vi "isMotorOn.vi"(1 "Device":refnum<k24>) -> (0 "isConnected":bool)   [LabVIEW 2014]
doc: "André Romero - 2017\nandretec@ifsc.usp.br"
uses:
  C:/UserLabs/Andre/LabView2014-32bits/kinesisTec/Kinesis/Thorlabs.MotionControl.TCube.DCServoCLI.dll
  Kinesis/Thorlabs.MotionControl.TCube.DCServoCLI.dll
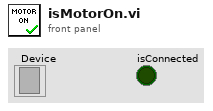
[diagram p1: front panel]
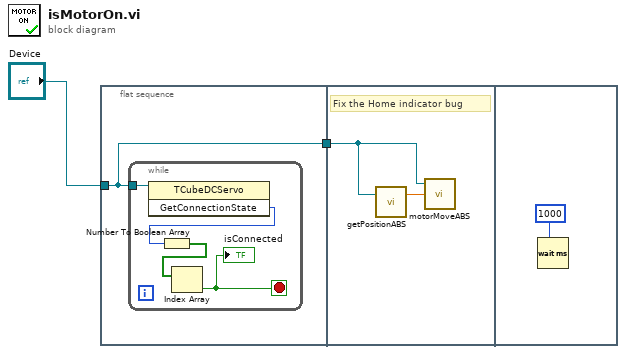
[diagram p0: block diagram]
diagram:
  n1 = flat-sequence {
    tunnel: "Device" -> [w3]
    tunnel: [w3] -> w1
    tunnel: w1 -> [w9]
    frame #0 {
      n2 = while {
        tunnel: w3 -> [w7]
        stop <- w4 stop-if-true
        n3 = invoke class="TCubeDCServo" method="GetConnectionState"(reference=w7) -> ("GetConnectionState"=w6:i32)  [unwired: 2 in, 2 out]
        n4 = Number To Boolean Array(number=w6) -> (Boolean array=w5:bool[])
        n5 = Index Array(array=w5) -> (element=w4:bool)  [unwired: 1 in]
        "isConnected" <- w4
      }
    }
    frame #1 {
      # "Fix the Home indicator bug"
      n6 = call "getPositionABS.vi"("Device"=w9) -> ("GetPOS"=w8:dbl)  [unwired: 2 in]
      n7 = call "motorMoveABS.vi"("position"=w8, "Device in"=w9) -> ()  [unwired: 3 in, 1 out]
    }
    frame #2 {
      n8 = Wait (ms)(milliseconds to wait=u32 1000) -> ()  [unwired: 1 out]
    }
  }
